vi "SentinelController v35 good v11.vi"() -> ()   [LabVIEW 2011]
uses:
  SC MT99XX tester states.ctl
  SC handler states.ctl
  Handler Types.ctl
  SC NS6040 tester states.ctl
  Echo tester states.ctl
  <vilib>/Instr/_visa.llb/Select Event Type.ctl
  <userlib>/configTool/configTool.llb/initConfigGlobal.vi
  <userlib>/configTool/configTool.llb/loadConfigFile.vi
  <userlib>/configTool/configTool.llb/closeConfig.vi
  <userlib>/configTool/configTool.llb/getProperty(DBL).vi
  <userlib>/configTool/configTool.llb/getProperty(U32).vi
  <userlib>/configTool/configTool.llb/getProperty(BOOL).vi
  <userlib>/configTool/configTool.llb/getProperty(I32).vi
  <userlib>/configTool/configTool.llb/getProperty(STR).vi
panel:
  out "Numeric 4":i32
  out "Numeric 3":i32
  out "Numeric 2":i32
  out "Numeric":i32
  out "H2 wt start hidden":u32
  out "H2 wt end hidden":u32
  out "H2 it start hidden":u32
  out "H2 it end hidden":u32
  out "H2 tt start hidden":u32
  out "H2 tt end hidden":u32
  in  "Data log path and filename":path=path "configuraitons/default_configuraiton.cfg"
  in  "Panels":T1(tab)=enum."System Configuration"
  in  "Test cell ID":string="default"
  in  "Operator name":string="default"
  in  "Lot number":string="default"
  in  "Configuration file path and filename":path
  in  "POWER":bool=TRUE
  in  "Tester Handler Config":T2=enum."Seiko-Epson NS6040" caption="Handler type"
  in  "H1 handler type":T2=enum."Seiko-Epson NS6040" caption="Handler type"
  in  "H2 handler type":T2=enum."Seiko-Epson NS6040" caption="Handler type"
  in  "H2 allow lower parallelism":bool
  in  "H1 allow lower parallelism":bool
  in  "H1 low yield warning":dbl=95.0 min=0.0 max=100.0 step=1.0
  in  "Ignore alarms until AFTER this many cycles":i32=20
  in  "H1 low yield alarm":dbl=85.0 min=0.0 max=100.0 step=1.0
  in  "H1 low UPH warning (%)":dbl=95.0 min=1.0 max=48000.0 step=1.0
  in  "H1 low UPH alarm (%)":dbl=90.0 min=1.0 max=48000.0 step=1.0
  in  "Enable data logging of all events":bool=TRUE
  in  "Enable electronic notification of alarms":bool
  in  "H2 low UPH alarm (%)":dbl=90.0 min=1.0 max=48000.0 step=1.0
  in  "H2 low UPH warning (%)":dbl=95.0 min=1.0 max=48000.0 step=1.0
  in  "H2 low yield alarm":dbl=90.0 min=0.0 max=100.0 step=1.0
  in  "H2  low yield warning":dbl=95.0 min=0.0 max=100.0 step=1.0
  in  "H1 enable halt\non yield alarm":bool
  in  "H2 enable halt\non yield alarm":bool
  in  "H1 enable halt\non UPH alarm":bool
  in  "H2 enable halt\non UPH alarm":bool
  out "H2 Device Count":u32 caption="Device Count"
  out "H1 Device Count":u32 caption="Decvice Count"
  out "H1 Good Units":u32 caption="Decvice Count"
  out "H2 Good Units":u32 caption="Device Count"
  out "H1 lot yield mon":dbl format="%.1f"
  out "H2 lot yield mon":dbl format="%.1f"
  out "UPH averaging":u32=20 min=2 max=100 step=1
  out "Yield averaging":u32=20 min=2 max=100 step=1
  in  "Push to reset charts":bool
  in  "Run":bool caption="Run / Stop"
  in  "Optimize handler speed":bool
  out "H1 parallelism":u32
  out "Utilization averaging":i32=6 min=2 max=20 step=1
  out "H2 nominal 2":bool=TRUE
  out "H2 warning 2":bool
  out "H2 alarm 2":bool
  out "H1 nominal 2":bool=TRUE
  out "H1 warning 2":bool
  out "H1 alarm 2":bool
  out "H2 nominal":bool=TRUE
  out "H2 warning":bool
  out "H2 alarm":bool
  out "H1 nominal":bool=TRUE
  out "H1 warning":bool
  out "H1 alarm":bool
  out "H2 Lock":bool
  out "H1 Lock":bool
  out "H2 measured Test Time":dbl caption="Index Time" format="%.2f"
  out "H2 measured  Index Time":dbl caption="Index Time" format="%.2f"
  out "H2 Indexing":bool
  out "H2 Testing":bool
  out "H2 Ready with sites":bool
  out "H2 On/Off-line":bool
  out "H2 measured Wait Time":dbl caption="Index Time" format="%.2f"
  out "H1 measured Test Time":dbl caption="Index Time" format="%.2f"
  out "H1 measured Index Time":dbl caption="Index Time" format="%.2f"
  out "H1 Indexing":bool
  out "H1 Testing":bool
  out "H1 Ready with sites":bool
  out "H1 On/Off-line":bool
  out "H1 measured Wait Time":dbl caption="Index Time" format="%.2f"
  out "System UPH":u32(knob) caption="Sys UPH" scale=0.0..30240.0 scale format="%#.0f"
  out "H2 UPH":cluster{u32, u32}(knob) scale=0.0..14400.0 scale format="%#.0f"
  out "H1 UPH":cluster{u32, u32}(knob) scale=0.0..14400.0 scale format="%#.0f"
  out "Sys utilization":dbl(knob) caption="Yield" scale=0.0..100.0
  in  "H2 online":bool=TRUE
  in  "H1 online":bool=TRUE
  in  "Tester online":bool=TRUE
  in  "Alert volume":u32(knob)=5 max=10 step=1 scale=0.0..10.0
  in  "Audio On / Off":bool
  out "SysUtilMon":cluster{i32, i32}(graph)
  out "H2 parallelism":u32 caption="H2 Paralellism"
  out "YieldMon":cluster{i32, i32, i32, i32}(graph)
  out "Program Parallelism":u32=8 caption="Tester Parallelism" min=1 max=16 step=1
  out "H2 calc UPH":dbl format="%#.0f"
  out "H1 Index Time 2":dbl caption="H1 index time"
  out "H1 Test Time 2":dbl caption="H1 test time"
  out "H1 P in formula":u32 caption="H1 Parallelism"
  out "H2 UPH per unit area":dbl format="%.1f"
  out "H1 calc UPH":dbl format="%#.0f"
  out "H1 UPH per unit area":dbl format="%.1f"
  out "Std mo cost ($/mo)":dbl
  out "Std unit cost\n(cents/device)":dbl format="%.3g"
  out "UPH":dbl format="%#.0f"
  in  "Hours per month":i32=730
  out "Std hourly\ncost ($/hr)":dbl format="%.2f"
  in  "Std cell \nfloorspace area":i32=200 min=10 max=1000 step=10
  in  "Overhead ($/mo)":dbl=1000.0 min=0.0 max=10000.0 step=100.0
  in  "Handler cost ($/mo)":dbl=2500.0 min=0.0 max=100000.0 step=100.0
  in  "Tester cost ($/mo)":dbl=8500.0 min=0.0 max=100000.0 step=500.0
  in  "Utilization (%)":u32=80 min=10 max=100 step=10
  out "Calendar days required\nfor testing all units":dbl format="%.1f"
  in  "# of devices to test":u32=10000000 min=1000 max=100000000 step=1000
  out "$ saved":i64 format="%#.0f"
  out "H2 IT (scycle)":dbl format="%.2f"
  out "H2 TT (s/cycle)":dbl format="%.2f"
  out "H2 WT (s/cycle)":dbl format="%.2f"
  out "H1 WT (s/cycle)":dbl format="%.2f"
  out "H1 IT (s/cycle)":dbl format="%.2f"
  out "H1 TT (s/cycle)":dbl format="%.2f"
  out "H2 units/cycle":u32 caption="H1 Parallelism"
  out "H1 units/cycle":u32
  out "Calc H1 UPH":u32
  out "Calc H2 UPH":u32
  out "Std cell floorspace area":i32
  out "Tandem unit cost\n(cents/device)":dbl format="%.3f"
  out "Hours per month 2":i32 caption="Hours per month"
  out "Total Mo Costs ($/mo) 3":dbl caption="Tandem mo cost ($/mo)"
  out "Total Mo Costs ($/mo) 2":dbl caption="Std mo cost ($/mo)"
  out "Calc\nsystem UPH":u32 caption="Simulated\nSystem UPH"
  out "Tandem\nfloorspace area":i32
  out "Tandem UPH\nper unit area":dbl format="%.1f"
  in  "Second handler cost ($/mo)":dbl=2500.0 min=0.0 max=10000.0 step=100.0
  out "Tandem hourly\ncost ($/hr)":dbl format="%.2f"
  in  "Celerint licensing cost ($/mo)":dbl=1000.0 min=0.0 max=10000.0 step=100.0
  in  "Celerint hardware cost ($/mo)":dbl min=0.0 max=10000.0 step=1.0
  in  "Additional floorspace\nfor second handler":i32=50 min=0 max=1000 step=10
  out "Number of text alerts":u32 caption="Number of alerts\nsent as notifications"
  in  "Enable text notification":bool
  out "Notifications Lot Display":string="default" caption="Lot number (not editable)"
  in  "Include\ndata log as\nattachment":bool=TRUE
  out "Number of email alerts":u32 caption="Number of alerts\nsent as notifications"
  out "Email alert - attachment (not editable)":path
  in  "Email alert - message":string="An alarm event has ocurred on a semiconductor test lot that you have requested to monitor.  Please see the attached data log for event details.\n\nThis message is generated automatically by the Sentinel Controller program.\n\nTo stop these messages, please contact the test floor operator and disable automatic alert notifictions.\n\n"
  in  "Email alert - engineer":string="harry@celerint.com"
  in  "Email alert - CC":string="hjr@celerint.com"
  in  "Enable email notification":bool
  in  "Carrier":enum16{"T-Mobile", "AT&T", "Verizon", "Sprint"}(ring)=enum."AT&T"
  in  "Phone number":string="5128263411"
  in  "Subject":string="From: Sentinel Controller"
  in  "Body":string="An alarm event has ocurred"
  in  "GPIB wait time (ms)":u32=1000
  in  "Slow for  Diagnostics":bool=TRUE
  out "GPIB bus 0 read error":bool
  out "GPIB Bus 0 traffic":string
  out "GPIB bus 1 traffic":string
  out "GPIB bus 2 traffic":string
  out "GPIB bus 0 write error":bool
  out "GPIB bus 1 read error":bool
  out "GPIB bus 1 write error":bool
  out "GPIB bus 2 write error":bool
  out "GPIB bus 2 read error":bool
  out "VISA bus 1 open error":bool
  out "VISA bus 2 open error":bool
  out "VISA bus 0 open error":bool
  out "VISA bus 0 close error":bool
  out "VISA bus 1 close error":bool
  out "VISA bus 2 close error":bool
  out "Decrease Handler Velocity":string
  out "Increase Handler Velocity":string
  out "Get Handler Velocity":string
  in  "SentCtrl listens to tester at":refnum<visa-resource-name>="GPIB0::INTFC"
  out "H2 Address":string
  out "H1 Address":string
  out "Tester address":string
  in  "SentCtrl talks to tester at":refnum<visa-resource-name>="GPIB0::0::INSTR"
  in  "SentCtrl listens to handler 1 at":refnum<visa-resource-name>="GPIB1::INTFC"
  in  "SentCtrl talks to handler 1 at":refnum<visa-resource-name>="GPIB1::1::INSTR"
  in  "SentCtrl listens to handler 2 at":refnum<visa-resource-name>="GPIB2::INTFC"
  in  "SentCtrl talks to handler 2 at":refnum<visa-resource-name>="GPIB2::1::INSTR"
  in  "Ni Logo":bool
  in  "Ni Logo 2":bool
  in  "Echo state of tester hid":T3
  in  "H1 echo hid":string
  in  "H2 echo hid":string
  in  "SRQ MASK from tester hid":string
  in  "H1 binning string hid":string
  in  "H2 binning string hid":string
  in  "H1 FULLSITES? response hid":string
  in  "H2 FULLSITES? response hid":string
  in  "H1 FULLSITES? binary hid":string
  in  "H2 FULLSITES? binary hid":string
  in  "H1 response to SPOLL hid":string
  in  "H2 response to SPOLL hid":string
  in  "H1 response to FR? hid":string
  in  "H2 response to FR? hid":string
  in  "NS6040 tester states H1 hid":T4
  in  "NS6040 tester states H2 hid":T4
  in  "MT99XX tester states H2 hid":T5
  in  "MT99XX tester states H1 hid":T5
  in  "GPIB parsed msg from tester hid":string
  in  "Message from H2 hid":string
  in  "Message from H1 hid":string
  in  "Message from tester hid":string
  in  "H1 response to *IDN? hid":string
  in  "H2 response to *IDN? hid":string
  in  "GPIB wait timeout hid":u32
  out "Number of data log entries hid":u32
  in  "Last locked handler hid":enum16{"H1", "H2"}(ring)
  out "SC measured wait time hid":dbl
  out "Exit SC tester H2 StMach hid":bool
  out "Exit SC tester H1 StMach hid":bool
  out "Exit SC handler StMach hid":bool
  out "H2 response to *HAND? hid":string
  out "H1 response to *HAND? hid":string
  in  "Tester loop counter hid":u32
  in  "H2 loop counter hid":u32
  in  "H1 loop counter hid":u32
  in  "Test Cycle State hid":T6(ring)
  in  "Test time expected hid":dbl
  out "H1 it end hidden":u32
  out "H1 wt start hidden":u32
  out "H1 tt start hidden":u32
  out "H1 wt end hidden":u32
  out "H1 tt end hidden":u32
  out "H1 it start hidden":u32
  in  "H1 SITES? response hid":string
  out "VISA bus 1 resource name out hid":refnum<visa-resource-name>
  out "VISA bus 1 error out hid":errorcluster
  out "VISA bus 2 error out hid":errorcluster
  out "VISA bus 2 resource name out hid":refnum<visa-resource-name>
  out "VISA bus 0 error out hid":errorcluster
  out "tester wt start hid":u32
  out "tester wt end hid":u32
  out "tester tt start hid":u32
  out "tester tt end hid":u32
  out "SC measured test time hid":dbl
  in  "Binning string from tester hid":string
  out "VISA bus 0 resource name out hid":refnum<visa-resource-name>
  in  "SC handler states hid":T7
  out "H1 Single Handler UPH hid":dbl
  out "H1 UPH warning limit hid":dbl
  out "H1 UPH alarm limit hid":dbl
  out "H2 Single Handler UPH hid":dbl
  out "H2 UPH warning limit hid":dbl
  out "H2 UPH alarm limit hid":dbl
  in  "Min Test Time hid":dbl=0.499 caption="Min Test Time" min=0.1 max=1.0 step=0.1 format="%#.1g"
  in  "H2 index time expected hid":dbl
  in  "H1 index time expected hid":dbl
  in  "system states hid":T8(ring)
  in  "system statuts hid":T9(ring)
  out "H1 cycle yield hid":dbl format="%.1f"
  out "H2 cycle yield hid":dbl format="%.1f"
  in  "H2 SITES? response hid":string
  # "Sentinel Controller\nfor\nTandlem Handler\nTest Cells \nwww.celerint.com"
  # "Turning off POWER will stop execution the Sentinel Controller Program"
  # "INPUT FILE"
  # "LOT INFORMATION"
  # "Celerint Sentinel Controller"
  # "SYSTEM SETTINGS"
  # "Tester Handler Config"
  # "Handler  1"
  # "Handler 2"
  # "Set UPH thresholds as % of max UPH"
  # "Set UPH thresholds as % of max UPH"
  # "test cycles (insertions)"
  # "Celerint Sentinel Controller"
  # "Handler 2"
  # "Handler 1"
  # "Yield"
  # "UPH"
  # "Yield"
  # "UPH"
  # "parallelism"
  # "lot yield (%)"
  # "good devices"
  # "devices tested"
  # "Data"
  # "Avg"
  # "wait time"
  # "index time"
  # "test time"
  # "waiting"
  # "H1"
  # "H2"
  # "testing"
  # "indexing"
  # "on/off-line"
  # "STANDARD SETUP"
  # "H2 calculated\nsimilarly"
  # "3600"
  # "Celerint Sentinel\nController Simulator"
  # "TANDEM HANDLER SETUP"
  # "SAVINGS"
  # "3600 (s/hr)"
  # "3600 (s/hr)"
  # "Celerint Sentinel Controller"
  # "Lot number will be appended automatically:"
  # "This data is read from the INI file (.cfg)\nat program start and is used to configure\nthe various GPIB interfaces on the Sentinel\nController."
  # "These setting are created based on the addresses read from the INI file."
  # "Laptop Tester Sim\nGPIB0,SC\naddress 0\nlisten at: GPIB0::INTFC\ntalk to: GPIB0::1::INSTR"
  # "*SITES?"
  # "binning"
  # "Bus 0"
  # "1011"
  # "SC\nGPIB0,Non-SC\naddress 1\nlisten at: GPIB0::INTFC\ntalk to: GPIB0::0::INSTR"
  # "SC\nGPIB1,SC\naddress 0\nlisten at: GPIB1::INTFC\ntalk to: GPIB1::0::INSTR"
  # "SC\nGPIB2,SC\naddress 0\nlisten at: GPIB2::INTFC\ntalk to: GPIB2::0::INSTR"
  # "NI PXI-1031"
  # "*SITES?"
  # "binning"
  # "*SITES?"
  # "binning"
  # "Bus 1"
  # "Bus 2"
  # "1011"
  # "1011"
  # "Laptop H1 Sim\nGPIB1,Non-SC\naddress 1\nlisten at: GPIB1::INTFC\ntalk to: GPIB1::0::INSTR"
  # "Laptop H2 Sim\nGPIB2,Non-SC\naddress 1\nlisten at: GPIB2::INTFC\ntalk to: GPIB2::0::INSTR"
  # "Note:\nUsually, there are default GPIB addresses used for the tester and handler.\nThese addresses are read in from the INI file (.cfrg extension) when this\nprogram initializes.  For the purposes of this map, we are using  these defaults:\n          - Semiconductor tester default GPIB address: 6\n          - Semiconductor handler default GPIB address: 14\nFor the purposes of this illustration, these addresses are purely arbitrary."
  # "Tester\nGPIB0,SC\naddress 6\nlisten at: GPIB0::INTFC\ntalk to: GPIB0:14::INSTR"
  # "*SITES?"
  # "binning"
  # "Bus 0"
  # "1011"
  # "SC\nGPIB0,Non-SC\naddress 14\nlisten at: GPIB1::INTFC\ntalk to: GPIB1:6::INSTR"
  # "SC\nGPIB1,SC\naddress 6\nlisten at: GPIB1::INTFC\ntalk to: GPIB1:14::INSTR"
  # "SC\nGPIB2,SC\naddress 6\nlisten at: GPIB2::INTFC\ntalk to: GPIB2:14::INSTR"
  # "NI PXI-1031"
  # "*SITES?"
  # "binning"
  # "*SITES?"
  # "binning"
  # "Bus 1"
  # "Bus 2"
  # "1011"
  # "1011"
  # "Handler 1\nGPIB0,Non-SC\naddress 14\nlisten at: GPIB0::INTFC\ntalk to: GPIB0:6::INSTR"
  # "Handler 2\nGPIB0,Non-SC\naddress 14\nlisten at: GPIB0::INTFC\ntalk to: GPIB0:6::INSTR"
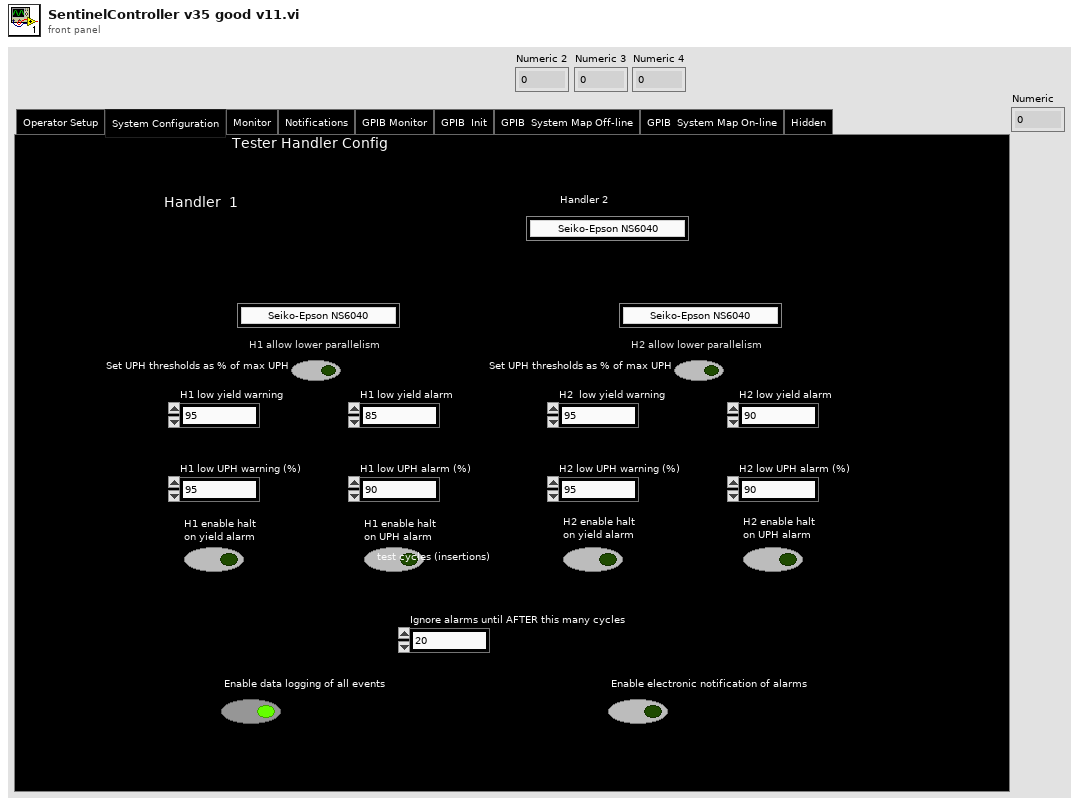
[diagram p1: front panel]
types:
  T1 = enum32{"Operator Setup", "System Configuration", "Monitor", "Benefit Analysis", "Notifications", "GPIB Monitor", "GPIB  Init", "GPIB  System Map Off-line", "GPIB  System Map On-line", "Hidden"}
  T2 = typedef "Handler Types.ctl" = enum16{"Multitest", "Seiko-Epson NS6040"}
  T3 = typedef "Echo tester states.ctl" = enum16{"ECHONG", "ECHOOK", "NO ECHO"}
  T4 = typedef "SC NS6040 tester states.ctl" = enum16{"initializing bus", "sending *IDN?", "serial polling handler", "sending Fullsites?", "testing", "sending BINON?", "sending ECHONG", "sending ECHOOK", "closing bus"}
  T5 = typedef "SC MT99XX tester states.ctl" = enum16{"initializing bus", "polling *SITES?", "sending *IDN?", "testing", "binning", "closing bus"}
  T6 = enum16{"idled", "SOT received", "SOT sent", "binning sent", "binning received", "sites ready received", "sites ready sent"}
  T7 = typedef "SC handler states.ctl" = enum16{"initializing bus", "waiting on event", "waiting on serial poll", "reading", "responding to *IDN?", "responding to Fullsites?", "responding to SITES?", "responding to HIDN?", "respond to HAND?", "testing", "responding to BINON", "responding to A BIN", "ECHONG", "ECHOOK", "responding to unknown command", "closing bus"}
  T8 = enum16{"H1 Ready", "H2 Ready", "No Handler Ready"}
  T9 = enum16{"H1NH2N", "H1NH2W", "H1NH2A", "H1WH2N", "H1WH2W", "H1WH2A", "H1AH2N", "H1AH2W", "H1AH2A"}
  T10 = enum16{"open", "replace", "create", "open or create", "replace or create", "replace or create with confirmation"}
  T11 = typedef "configRef.ctl" = refnum<vi>
  T12 = cluster{i32, "rolling avg out":dbl, "H1 low yield alarm":dbl, "H2 low yield alarm":dbl}
  T13 = cluster{"rolling avg out":dbl, i32, "H1 low yield alarm":dbl, "H2 low yield alarm":dbl}
  T14 = typedef "Select Event Type.ctl" = u32
diagram:
  n1 = flat-sequence {
    frame #0 {
      # "This frame contains ALL declarations for control and indicators.\nAll hidden objects are on frame #9.  On the front panel, these hidden\nobjects are located on a tab that is hidden."
      n2 = stacked-sequence {
        frame #0 {
        }
        frame #1 {
          # "Operator Setup Tab"
        }
        frame #2 {
          # "System Config Tab"
        }
        frame #3 {
          w2 = FALSE ("H2 Testing")
          w1 = FALSE ("H1 Testing")
          # "Monitor Tab"
          n3 = local write "Run"(FALSE ("Run")) -> ()
          "H1 Testing" <- w1
          "H1 Ready with sites" <- w1
          "H1 Indexing" <- w1
          "H2 Testing" <- w2
          "H2 Ready with sites" <- w2
          "H2 Indexing" <- w2
          "H2 Good Units" <- 0
          "H2 Device Count" <- 0
          "H2 lot yield mon" <- 100.0 ("H2 Yield  Mon")
          "H1 lot yield mon" <- 100.0 ("H1 Yield Mon")
          "H1 Good Units" <- u32 0
          "H1 Device Count" <- u32 0
        }
        frame #4 {
          # "Benefits Tab"
        }
        frame #5 {
          # "Notifications"
        }
        frame #6 {
          # "GPIB Monitor"
          n4 = local write "Slow for  Diagnostics"(FALSE ("Slow for  Diagnostics")) -> ()
          n5 = local write "GPIB wait time (ms)"(u32 1000 ("GPIB wait time (ms)")) -> ()
        }
        frame #7 {
          # "GPIB Init"
        }
        frame #8 {
          # "GPIB System Maps - Bothg off-line and on-line combined"
        }
        frame #9 {
          (unwired) 0.031 ("tester measured wait time")
          # "Hidden controls and indicators"
          n6 = local write "Last locked handler hid"(enum16{"H1", "H2"}."H1" ("Last locked handler")) -> ()
          "SC measured test time hid" <- 1.0 ("tester measured test time")
          "H1 response to *HAND? hid" <- "" ("H1 response to *HAND? hidden")
          "H2 response to *HAND? hid" <- "" ("H2 response to *HAND? hidden")
          "Exit SC handler StMach hid" <- FALSE ("Exit tester state machine")
          "Exit SC tester H1 StMach hid" <- FALSE ("Exit H1 state machine")
          "Exit SC tester H2 StMach hid" <- FALSE ("Exit H2 state machine")
          "SC measured wait time hid" <- 1.0 ("tester measured wait time hid")
          "H2 cycle yield hid" <- 100.0 ("H2 Yield  Mon")
          "H1 cycle yield hid" <- 100.0 ("H1 Yield Mon")
        }
      }
    }
    frame #1 {
      n7 = local write "POWER"(TRUE ("POWER")) -> ()
    }
    frame #2 {
      # "This frame handles verifying that the configuration file exists and is valaid.\nIt also creates the data log."
      n8 = local read "Configuration file path and filename"() -> (w25:path)
      n9 = call <vilib>:"Application Directory.vi"() -> ("Application Directory"=w27:path)
      n10 = Equal?(x=w25, y=path "") -> (x = y?=w24:bool)
      n11 = Get Date/Time String(want seconds? (F)=TRUE) -> (date string=w40:string, time string=w32:string)  [unwired: 2 in]
      n12 = Build Path(base path=w27, name or relative path="datalogs") -> (appended path=w45:path)
      n13 = Path To String(path=w45) -> (string=w36:string)
      n14 = Search and Replace String(replace all?=TRUE ("replace all? (F)"), input string=w40, search string="/", replace string="-" ("replace string (\"\")")) -> (result string=w30:string)  [unwired: 4 in, 3 out]
      n15 = Search and Replace String(replace all?=TRUE ("replace all? (F)"), input string=w32, search string=":", replace string="." ("replace string (\"\")")) -> (result string=w31:string)  [unwired: 4 in, 3 out]
      n16 = case shown="True" w24 {
        tunnel: w25 -> [w47 _]
        frame False {
          n17 = call <vilib>:"Check if File or Folder Exists.vi"("path"=w47) -> ("file or folder exists?"=w46:bool)  [unwired: 8 in, 2 out]
          n18 = case shown="False" w46 {
            frame False {
              n19 = local write "POWER"(FALSE ("POWER")) -> ()
              n20 = One Button Dialog(message="Fatal error 100: \nConfiguration file does not exist!", button name ("OK")="Dismiss and Restart") -> ()  [unwired: 1 out]
            }
            frame True {
              n21 = local read "Configuration file path and filename"() -> (w54:path)
              n22 = call-poly <userlib>:"manageConfig.vi"() -> ("config ref out"=w55:T11)  [unwired: 10 in, 1 out]
              n23 = call-poly <userlib>:"manageConfig.vi"("access (0:read/write)"=enum16{"read/write", "read-only", "write-only"}."read-only", "config file path"=w54, "config ref"=w55) -> ("error out"=w53:errorcluster, "config ref out"=w51:T11)  [unwired: 6 in, 1 out]
              n24 = Unbundle By Name(w53) -> ("status"=w52:bool)
              n25 = call-poly <userlib>:"manageConfig.vi"("config ref"=w51) -> ()  [unwired: 10 in, 1 out]
              n26 = case shown="True" w52 {
                frame False {
                }
                frame True {
                  n27 = local write "POWER"(FALSE ("POWER")) -> ()
                  n28 = One Button Dialog(message="Fatal error 101:\nConfiguration file is corrupted\nor is not a compliant format!", button name ("OK")="Dismiss and Restart") -> ()  [unwired: 1 out]
                }
              }
            }
          }
        }
        frame True {
          n29 = call <vilib>:"Application Directory.vi"() -> ("Application Directory"=w63:path)
          n30 = Build Path(base path=w63, name or relative path="configurations") -> (appended path=w60:path)
          n31 = Path To String(path=w60) -> (string=w65:string)
          n32 = Concatenate Strings(w65, "\\" ("string"), "default_configuration.cfg" ("string")) -> (w66:string)
          n33 = String To Path(string=w66) -> (path=w67:path)
          n34 = local write "Configuration file path and filename"(w67) -> ()
        }
      }
      n35 = Concatenate Strings(w36, "\\" ("string"), w30, " " ("string"), w31, ".txt" ("string")) -> (w42:string)
      n36 = String To Path(string=w42) -> (path=w44:path)
      n37 = local write "Data log path and filename"(w44) -> ()
    }
    frame #3 {
      # "This frame reads the INI file and initializes all data that is under engineering control."
      n38 = local read "POWER"() -> (w68:bool)
      n39 = case shown="True" w68 {
        frame False {
        }
        frame True {
          n40 = stacked-sequence {
            frame #0 {
              # "Load data from the INI file for the System Configuration tab"
              n41 = local read "Configuration file path and filename"() -> (w162:path)
              n42 = call-poly <userlib>:"manageConfig.vi"() -> ("config ref out"=w163:T11)  [unwired: 10 in, 1 out]
              n43 = call-poly <userlib>:"manageConfig.vi"("access (0:read/write)"=enum16{"read/write", "read-only", "write-only"}."read-only", "config file path"=w162, "config ref"=w163) -> ("error out"=w101:errorcluster, "config ref out"=w100:T11)  [unwired: 6 in, 1 out]
              n44 = call-poly <userlib>:"manageConfig.vi"("error in"=w101, "property path"="SCS.SimCfgCtrls.Test time expected" ("key"), "config ref"=w100) -> ("error out"=w97:errorcluster, "data"=w103:dbl, "config ref out"=w104:T11)  [unwired: 5 in, 1 out]
              n45 = local write "Test time expected hid"(w103) -> ()
              n46 = call-poly <userlib>:"manageConfig.vi"("error in"=w97, "property path"="SCS.SimCfgCtrls.H1 Parallelism", "config ref"=w104) -> ("error out"=w96:errorcluster, "value"=w116:u32, "config ref out"=w110:T11)  [unwired: 5 in, 1 out]
              n47 = local write "H1 parallelism"(w116) -> ()
              n48 = call-poly <userlib>:"manageConfig.vi"("error in"=w96, "property path"="SCS.SimCfgCtrls.H2 Parallelism", "config ref"=w110) -> ("error out"=w95:errorcluster, "value"=w112:u32, "config ref out"=w109:T11)  [unwired: 5 in, 1 out]
              n49 = local write "H2 parallelism"(w112) -> ()
              n50 = call-poly <userlib>:"manageConfig.vi"("error in"=w95, "property path"="SCS.SimCfgCtrls.Program Parallelism", "config ref"=w109) -> ("error out"=w94:errorcluster, "value"=w111:u32, "config ref out"=w102:T11)  [unwired: 5 in, 1 out]
              n51 = local write "Program Parallelism"(w111) -> ()
              n52 = call-poly <userlib>:"manageConfig.vi"("error in"=w94, "property path"="SCS.SimCfgCtrls.H1 index time expected", "config ref"=w102) -> ("error out"=w93:errorcluster, "data"=w106:dbl, "config ref out"=w115:T11)  [unwired: 5 in, 1 out]
              n53 = local write "H1 index time expected hid"(w106) -> ()
              n54 = call-poly <userlib>:"manageConfig.vi"("error in"=w93, "property path"="SCS.SimCfgCtrls.H2 index time expected", "config ref"=w115) -> ("error out"=w99:errorcluster, "data"=w105:dbl, "config ref out"=w98:T11)  [unwired: 5 in, 1 out]
              n55 = local write "H2 index time expected hid"(w105) -> ()
              n56 = call-poly <userlib>:"manageConfig.vi"("error in"=w99, "property path"="SCS.SimCfgCtrls.H1 low yield warning" ("key"), "config ref"=w98) -> ("error out"=w92:errorcluster, "data"=w139:dbl, "config ref out"=w149:T11)  [unwired: 5 in, 1 out]
              n57 = local write "H1 low yield warning"(w139) -> ()
              n58 = call-poly <userlib>:"manageConfig.vi"("error in"=w92, "property path"="SCS.SimCfgCtrls.H1 low yield alarm", "config ref"=w149) -> ("error out"=w91:errorcluster, "data"=w138:dbl, "config ref out"=w148:T11)  [unwired: 5 in, 1 out]
              n59 = local write "H1 low yield alarm"(w138) -> ()
              n60 = call-poly <userlib>:"manageConfig.vi"("error in"=w91, "property path"="SCS.SimCfgCtrls.H1 low UPH warning (%)", "config ref"=w148) -> ("error out"=w90:errorcluster, "data"=w137:dbl, "config ref out"=w150:T11)  [unwired: 5 in, 1 out]
              n61 = local write "H1 low UPH warning (%)"(w137) -> ()
              n62 = call-poly <userlib>:"manageConfig.vi"("error in"=w90, "property path"="SCS.SimCfgCtrls.H1 low UPH alarm (%)", "config ref"=w150) -> ("error out"=w89:errorcluster, "data"=w136:dbl, "config ref out"=w151:T11)  [unwired: 5 in, 1 out]
              n63 = local write "H1 low UPH alarm (%)"(w136) -> ()
              n64 = call-poly <userlib>:"manageConfig.vi"("error in"=w89, "property path"="SCS.SimCfgCtrls.H1 enable halt on yield alarm", "config ref"=w151) -> ("error out"=w88:errorcluster, "value"=w135:bool, "config ref out"=w152:T11)  [unwired: 5 in, 1 out]
              n65 = local write "H1 enable halt\non yield alarm"(w135) -> ()
              n66 = call-poly <userlib>:"manageConfig.vi"("error in"=w88, "property path"="SCS.SimCfgCtrls.H1 enable halt on UPH alarm", "config ref"=w152) -> ("error out"=w87:errorcluster, "value"=w134:bool, "config ref out"=w153:T11)  [unwired: 5 in, 1 out]
              n67 = local write "H1 enable halt\non UPH alarm"(w134) -> ()
              n68 = call-poly <userlib>:"manageConfig.vi"("error in"=w87, "property path"="SCS.SimCfgCtrls.H2 low yield warning", "config ref"=w153) -> ("error out"=w86:errorcluster, "data"=w133:dbl, "config ref out"=w154:T11)  [unwired: 5 in, 1 out]
              n69 = local write "H2  low yield warning"(w133) -> ()
              n70 = call-poly <userlib>:"manageConfig.vi"("error in"=w86, "property path"="SCS.SimCfgCtrls.H2 low yield alarm", "config ref"=w154) -> ("error out"=w85:errorcluster, "data"=w132:dbl, "config ref out"=w155:T11)  [unwired: 5 in, 1 out]
              n71 = local write "H2 low yield alarm"(w132) -> ()
              n72 = call-poly <userlib>:"manageConfig.vi"("error in"=w85, "property path"="SCS.SimCfgCtrls.H2 low UPH warning (%)", "config ref"=w155) -> ("error out"=w84:errorcluster, "data"=w131:dbl, "config ref out"=w123:T11)  [unwired: 5 in, 1 out]
              n73 = local write "H2 low UPH warning (%)"(w131) -> ()
              n74 = call-poly <userlib>:"manageConfig.vi"("error in"=w84, "property path"="SCS.SimCfgCtrls.H2 low UPH alarm (%)", "config ref"=w123) -> ("error out"=w83:errorcluster, "data"=w121:dbl, "config ref out"=w122:T11)  [unwired: 5 in, 1 out]
              n75 = local write "H2 low UPH alarm (%)"(w121) -> ()
              n76 = call-poly <userlib>:"manageConfig.vi"("error in"=w83, "property path"="SCS.SimCfgCtrls.H2 enable halt on yield alarm", "config ref"=w122) -> ("error out"=w82:errorcluster, "value"=w130:bool, "config ref out"=w156:T11)  [unwired: 5 in, 1 out]
              n77 = local write "H2 enable halt\non yield alarm"(w130) -> ()
              n78 = call-poly <userlib>:"manageConfig.vi"("error in"=w82, "property path"="SCS.SimCfgCtrls.H2 enable halt on UPH alarm", "config ref"=w156) -> ("error out"=w81:errorcluster, "value"=w129:bool, "config ref out"=w120:T11)  [unwired: 5 in, 1 out]
              n79 = local write "H2 enable halt\non UPH alarm"(w129) -> ()
              n80 = call-poly <userlib>:"manageConfig.vi"("error in"=w81, "property path"="SCS.SimCfgCtrls.Ignore alarms until this many cycles", "config ref"=w120) -> ("error out"=w80:errorcluster, "value"=w128:i32, "config ref out"=w119:T11)  [unwired: 5 in, 1 out]
              n81 = local write "Ignore alarms until AFTER this many cycles"(w128) -> ()
              n82 = call-poly <userlib>:"manageConfig.vi"("error in"=w80, "property path"="SCS.SimCfgCtrls.Enable data logging", "config ref"=w119) -> ("error out"=w79:errorcluster, "value"=w127:bool, "config ref out"=w140:T11)  [unwired: 5 in, 1 out]
              n83 = local write "Enable data logging of all events"(w127) -> ()
              n84 = call-poly <userlib>:"manageConfig.vi"("error in"=w79, "property path"="SCS.SimCfgCtrls.Enable electronic notification of alarms", "config ref"=w140) -> ("error out"=w78:errorcluster, "value"=w126:bool, "config ref out"=w76:T11)  [unwired: 5 in, 1 out]
              n85 = local write "Enable electronic notification of alarms"(w126) -> ()
              n86 = call-poly <userlib>:"manageConfig.vi"("error in"=w78, "property path"="SCS.SimCfgCtrls.H1 allow lower parallelism", "config ref"=w76) -> ("error out"=w77:errorcluster, "value"=w70:bool, "config ref out"=w75:T11)  [unwired: 5 in, 1 out]
              n87 = local write "H1 allow lower parallelism"(w70) -> ()
              n88 = call-poly <userlib>:"manageConfig.vi"("error in"=w77, "property path"="SCS.SimCfgCtrls.H2 allow lower parallelism", "config ref"=w75) -> ("error out"=w73:errorcluster, "value"=w69:bool, "config ref out"=w74:T11)  [unwired: 5 in, 1 out]
              n89 = local write "H2 allow lower parallelism"(w69) -> ()
              n90 = call-poly <userlib>:"manageConfig.vi"("error in (no error)"=w73, "config ref"=w74) -> ()  [unwired: 9 in, 1 out]
            }
            frame #1 {
              # "Load data from the INI file for the Monitor tab"
              n91 = local read "Configuration file path and filename"() -> (w201:path)
              n92 = call-poly <userlib>:"manageConfig.vi"() -> ("error out"=w175:errorcluster, "config ref out"=w202:T11)  [unwired: 10 in]
              n93 = call-poly <userlib>:"manageConfig.vi"("error in (no error)"=w175, "access (0:read/write)"=enum16{"read/write", "read-only", "write-only"}."read-only", "config file path"=w201, "config ref"=w202) -> ("error out"=w204:errorcluster, "config ref out"=w206:T11)  [unwired: 5 in, 1 out]
              n94 = call-poly <userlib>:"manageConfig.vi"("error in"=w204, "property path"="SCS.Monitor.Optimize handler speed" ("key"), "config ref"=w206) -> ("error out"=w174:errorcluster, "value"=w184:bool, "config ref out"=w176:T11)  [unwired: 5 in, 1 out]
              n95 = local write "Optimize handler speed"(w184) -> ()
              n96 = call-poly <userlib>:"manageConfig.vi"("error in"=w174, "property path"="SCS.Monitor.Tester on-line" ("key"), "config ref"=w176) -> ("error out"=w173:errorcluster, "value"=w183:bool, "config ref out"=w197:T11)  [unwired: 5 in, 1 out]
              n97 = local write "Tester online"(w183) -> ()
              n98 = call-poly <userlib>:"manageConfig.vi"("error in"=w173, "property path"="SCS.Monitor.H1 on-line" ("key"), "config ref"=w197) -> ("error out"=w172:errorcluster, "value"=w182:bool, "config ref out"=w196:T11)  [unwired: 5 in, 1 out]
              n99 = local write "H1 online"(w182) -> ()
              n100 = call-poly <userlib>:"manageConfig.vi"("error in"=w172, "property path"="SCS.Monitor.H2 on-line" ("key"), "config ref"=w196) -> ("error out"=w171:errorcluster, "value"=w181:bool, "config ref out"=w195:T11)  [unwired: 5 in, 1 out]
              n101 = local write "H2 online"(w181) -> ()
              n102 = call-poly <userlib>:"manageConfig.vi"("error in"=w171, "property path"="SCS.Monitor.Utilization averaging", "config ref"=w195) -> ("error out"=w170:errorcluster, "value"=w177:i32, "config ref out"=w194:T11)  [unwired: 5 in, 1 out]
              n103 = local write "Utilization averaging"(w177) -> ()
              n104 = call-poly <userlib>:"manageConfig.vi"("error in"=w170, "property path"="SCS.Monitor.Audio On/Off", "config ref"=w194) -> ("error out"=w169:errorcluster, "config ref out"=w193:T11)  [unwired: 5 in, 2 out]
              n105 = call-poly <userlib>:"manageConfig.vi"("error in"=w169, "property path"="SCS.Monitor.Alert volume", "config ref"=w193) -> ("error out"=w168:errorcluster, "value"=w180:u32, "config ref out"=w192:T11)  [unwired: 5 in, 1 out]
              n106 = local write "Alert volume"(w180) -> ()
              n107 = call-poly <userlib>:"manageConfig.vi"("error in"=w168, "property path"="SCS.Monitor.UPH averaging", "config ref"=w192) -> ("error out"=w167:errorcluster, "value"=w179:u32, "config ref out"=w191:T11)  [unwired: 5 in, 1 out]
              n108 = local write "UPH averaging"(w179) -> ()
              n109 = call-poly <userlib>:"manageConfig.vi"("error in"=w167, "property path"="SCS.Monitor.Yield averaging", "config ref"=w191) -> ("error out"=w166:errorcluster, "value"=w178:u32, "config ref out"=w190:T11)  [unwired: 5 in, 1 out]
              n110 = local write "Yield averaging"(w178) -> ()
              n111 = call-poly <userlib>:"manageConfig.vi"("error in (no error)"=w166, "config ref"=w190) -> ()  [unwired: 9 in, 1 out]
            }
            frame #2 {
              # "Load data from the INI file for the Benefits tab"
              n112 = local read "Configuration file path and filename"() -> (w243:path)
              n113 = call-poly <userlib>:"manageConfig.vi"() -> ("error out"=w216:errorcluster, "config ref out"=w244:T11)  [unwired: 10 in]
              n114 = call-poly <userlib>:"manageConfig.vi"("error in (no error)"=w216, "access (0:read/write)"=enum16{"read/write", "read-only", "write-only"}."read-only", "config file path"=w243, "config ref"=w244) -> ("error out"=w246:errorcluster, "config ref out"=w248:T11)  [unwired: 5 in, 1 out]
              n115 = call-poly <userlib>:"manageConfig.vi"("error in"=w246, "property path"="SCS.Benefits.Tester cost" ("key"), "config ref"=w248) -> ("error out"=w215:errorcluster, "data"=w234:dbl, "config ref out"=w225:T11)  [unwired: 5 in, 1 out]
              n116 = local write "Tester cost ($/mo)"(w234) -> ()
              n117 = call-poly <userlib>:"manageConfig.vi"("error in"=w215, "property path"="SCS.Benefits.Handler cost" ("key"), "config ref"=w225) -> ("error out"=w214:errorcluster, "data"=w233:dbl, "config ref out"=w224:T11)  [unwired: 5 in, 1 out]
              n118 = local write "Handler cost ($/mo)"(w233) -> ()
              n119 = call-poly <userlib>:"manageConfig.vi"("error in"=w214, "property path"="SCS.Benefits.Test cell overhead" ("key"), "config ref"=w224) -> ("error out"=w213:errorcluster, "data"=w232:dbl, "config ref out"=w223:T11)  [unwired: 5 in, 1 out]
              n120 = local write "Overhead ($/mo)"(w232) -> ()
              n121 = call-poly <userlib>:"manageConfig.vi"("error in"=w213, "property path"="SCS.Benefits.Hours per month" ("key"), "config ref"=w223) -> ("error out"=w212:errorcluster, "value"=w231:i32, "config ref out"=w222:T11)  [unwired: 5 in, 1 out]
              n122 = local write "Hours per month"(w231) -> ()
              n123 = call-poly <userlib>:"manageConfig.vi"("error in"=w212, "property path"="SCS.Benefits.STD cell floorspace area" ("key"), "config ref"=w222) -> ("error out"=w211:errorcluster, "value"=w230:i32, "config ref out"=w221:T11)  [unwired: 5 in, 1 out]
              n124 = local write "Std cell \nfloorspace area"(w230) -> ()
              n125 = call-poly <userlib>:"manageConfig.vi"("error in"=w211, "property path"="SCS.Benefits.Celerint hardware cost" ("key"), "config ref"=w221) -> ("error out"=w210:errorcluster, "data"=w229:dbl, "config ref out"=w220:T11)  [unwired: 5 in, 1 out]
              n126 = local write "Celerint hardware cost ($/mo)"(w229) -> ()
              n127 = call-poly <userlib>:"manageConfig.vi"("error in"=w210, "property path"="SCS.Benefits.Celerint licensing cost" ("key"), "config ref"=w220) -> ("error out"=w209:errorcluster, "data"=w228:dbl, "config ref out"=w219:T11)  [unwired: 5 in, 1 out]
              n128 = local write "Celerint licensing cost ($/mo)"(w228) -> ()
              n129 = call-poly <userlib>:"manageConfig.vi"("error in"=w209, "property path"="SCS.Benefits.Second handler cost" ("key"), "config ref"=w219) -> ("error out"=w208:errorcluster, "data"=w227:dbl, "config ref out"=w218:T11)  [unwired: 5 in, 1 out]
              n130 = local write "Second handler cost ($/mo)"(w227) -> ()
              n131 = call-poly <userlib>:"manageConfig.vi"("error in"=w208, "property path"="SCS.Benefits.Additional floorspace for seconed handler" ("key"), "config ref"=w218) -> ("error out"=w207:errorcluster, "value"=w226:i32, "config ref out"=w217:T11)  [unwired: 5 in, 1 out]
              n132 = local write "Additional floorspace\nfor second handler"(w226) -> ()
              n133 = call-poly <userlib>:"manageConfig.vi"("error in (no error)"=w207, "config ref"=w217) -> ()  [unwired: 9 in, 1 out]
            }
            frame #3 {
              w259 = "SCS.Notification.Enable text notification"  # key
              w265 = "SCS.Notification.Phone Number"  # key
              w266 = "SCS.Notification.Enable email notification"  # key
              w273 = "SCS.Notification.Email alert - Engineer"  # key
              # "Load data from the INI file for the Benefits tab"
              n134 = local read "Configuration file path and filename"() -> (w270:path)
              n135 = call-poly <userlib>:"manageConfig.vi"() -> ("error out"=w255:errorcluster, "config ref out"=w271:T11)  [unwired: 10 in]
              n136 = call-poly <userlib>:"manageConfig.vi"("error in (no error)"=w255, "access (0:read/write)"=enum16{"read/write", "read-only", "write-only"}."read-only", "config file path"=w270, "config ref"=w271) -> ("error out"=w254:errorcluster, "config ref out"=w274:T11)  [unwired: 5 in, 1 out]
              n137 = call-poly <userlib>:"manageConfig.vi"("error in"=w254, "property path"=w273, "config ref"=w274) -> ("error out"=w253:errorcluster, "value"=w268:string, "config ref out"=w264:T11)  [unwired: 5 in, 1 out]
              n138 = local write "Email alert - engineer"(w268) -> ()
              n139 = call-poly <userlib>:"manageConfig.vi"("error in"=w253, "property path"="SCS.Notification.Email alert CC", "config ref"=w264) -> ("error out"=w252:errorcluster, "value"=w267:string, "config ref out"=w263:T11)  [unwired: 5 in, 1 out]
              n140 = local write "Email alert - CC"(w267) -> ()
              n141 = call-poly <userlib>:"manageConfig.vi"("error in"=w252, "property path"=w266, "config ref"=w263) -> ("error out"=w251:errorcluster, "value"=w261:bool, "config ref out"=w258:T11)  [unwired: 5 in, 1 out]
              n142 = local write "Enable email notification"(w261) -> ()
              n143 = call-poly <userlib>:"manageConfig.vi"("error in"=w251, "property path"=w259, "config ref"=w258) -> ("error out"=w250:errorcluster, "value"=w256:bool, "config ref out"=w257:T11)  [unwired: 5 in, 1 out]
              n144 = local write "Enable text notification"(w256) -> ()
              n145 = call-poly <userlib>:"manageConfig.vi"("error in"=w250, "property path"=w265, "config ref"=w257) -> ("error out"=w249:errorcluster, "value"=w260:string, "config ref out"=w262:T11)  [unwired: 5 in, 1 out]
              n146 = local write "Phone number"(w260) -> ()
              n147 = call-poly <userlib>:"manageConfig.vi"("error in (no error)"=w249, "config ref"=w262) -> ()  [unwired: 9 in, 1 out]
            }
            frame #4 {
              # "This reads the GPIB addresses and related command from the INI file (.cfg)"
              n148 = local read "Configuration file path and filename"() -> (w301:path)
              n149 = call-poly <userlib>:"manageConfig.vi"() -> ("config ref out"=w302:T11)  [unwired: 10 in, 1 out]
              n150 = call-poly <userlib>:"manageConfig.vi"("access (0:read/write)"=enum16{"read/write", "read-only", "write-only"}."read-only", "config file path"=w301, "config ref"=w302) -> ("error out"=w304:errorcluster, "config ref out"=w306:T11)  [unwired: 6 in, 1 out]
              n151 = call-poly <userlib>:"manageConfig.vi"("error in"=w304, "property path"="SCS.GPIB.Tester Address" ("key"), "config ref"=w306) -> ("error out"=w291:errorcluster, "value"=w283:string, "config ref out"=w297:T11)  [unwired: 5 in, 1 out]
              n152 = local write "Tester address"(w283) -> ()
              n153 = call-poly <userlib>:"manageConfig.vi"("error in"=w291, "property path"="SCS.GPIB.H1 Address" ("key"), "config ref"=w297) -> ("error out"=w290:errorcluster, "value"=w282:string, "config ref out"=w296:T11)  [unwired: 5 in, 1 out]
              n154 = local write "H1 Address"(w282) -> ()
              n155 = call-poly <userlib>:"manageConfig.vi"("error in"=w290, "property path"="SCS.GPIB.H2 Address" ("key"), "config ref"=w296) -> ("error out"=w289:errorcluster, "value"=w281:string, "config ref out"=w295:T11)  [unwired: 5 in, 1 out]
              n156 = local write "H2 Address"(w281) -> ()
              n157 = call-poly <userlib>:"manageConfig.vi"("error in"=w289, "property path"="SCS.GPIB.SOT" ("key"), "config ref"=w295) -> ("error out"=w288:errorcluster, "config ref out"=w277:T11)  [unwired: 5 in, 2 out]
              n158 = call-poly <userlib>:"manageConfig.vi"("error in"=w288, "property path"="SCS.GPIB.Get Handler Velocity" ("key"), "config ref"=w277) -> ("error out"=w287:errorcluster, "value"=w280:string, "config ref out"=w276:T11)  [unwired: 5 in, 1 out]
              n159 = local write "Get Handler Velocity"(w280) -> ()
              n160 = call-poly <userlib>:"manageConfig.vi"("error in"=w287, "property path"="SCS.GPIB.Increase Handler Velocity" ("key"), "config ref"=w276) -> ("error out"=w286:errorcluster, "value"=w279:string, "config ref out"=w275:T11)  [unwired: 5 in, 1 out]
              n161 = local write "Increase Handler Velocity"(w279) -> ()
              n162 = call-poly <userlib>:"manageConfig.vi"("error in"=w286, "property path"="SCS.GPIB.Decrease Handler Velocity" ("key"), "config ref"=w275) -> ("error out"=w285:errorcluster, "value"=w278:string, "config ref out"=w284:T11)  [unwired: 5 in, 1 out]
              n163 = local write "Decrease Handler Velocity"(w278) -> ()
              n164 = call-poly <userlib>:"manageConfig.vi"("error in (no error)"=w285, "config ref"=w284) -> ()  [unwired: 9 in, 1 out]
            }
          }
        }
      }
    }
    frame #4 {
      # "This frame writes the headewr to the data log.\nIt includes setup and configuration information for the lot."
      n165 = local read "POWER"() -> (w307:bool)
      n166 = case shown="True" w307 {
        frame False {
        }
        frame True {
          w313 = "\r\n"
          n167 = local read "Lot number"() -> (w317:string)
          n168 = local read "Test cell ID"() -> (w315:string)
          n169 = local read "H1 online"() -> (w325:bool)
          n170 = local read "H2 online"() -> (w326:bool)
          n171 = local read "Data log path and filename"() -> (w308:path)
          n172 = local read "Operator name"() -> (w319:string)
          n173 = local read "H1 UPH warning limit hid"() -> (w321:dbl)
          n174 = local read "H2 UPH warning limit hid"() -> (w323:dbl)
          n175 = local read "H2  low yield warning"() -> (w322:dbl)
          n176 = local read "H1 low yield warning"() -> (w320:dbl)
          n177 = case shown="True" w325 {
            tunnel: ["H1 Off-Line" "H1 On-Line"] -> w327
            frame False {
            }
            frame True {
            }
          }
          n178 = case shown="True" w326 {
            tunnel: ["H2 Off-Line" "H2 On-Line"] -> w332
            frame False {
            }
            frame True {
            }
          }
          n179 = local write "Email alert - attachment (not editable)"(w308) -> ()
          n180 = Number To Decimal String(number=w320) -> (decimal integer string=w329:string)  [unwired: 1 in]
          n181 = Number To Decimal String(number=w321) -> (decimal integer string=w331:string)  [unwired: 1 in]
          n182 = Number To Decimal String(number=w322) -> (decimal integer string=w334:string)  [unwired: 1 in]
          n183 = Number To Decimal String(number=w323) -> (decimal integer string=w336:string)  [unwired: 1 in]
          n184 = Get Date/Time String() -> (date string=w310:string, time string=w312:string)  [unwired: 3 in]
          n185 = Concatenate Strings(w310, "   " ("string"), w312, w313, "Test Cell ID: ", w315, w313, "Lot Number: ", w317, w313, "Operator Name:  ", w319, w313, "System Started", w313, w327, w313, "H1 Low Yield Warning Limit: ", w329, w313, "H1 Low UPH Warning Limit: ", w331, w313, w332, w313, "H2 Low Yield Warning Limit: ", w334, w313, "H2 Low UPH Warning Limit: ", w336, w313, w313) -> (w337:string)
          n186 = call "SentinelDatalog.vi"("operation (0:open)"=T10."open or create", "String"=w337, "data log path"=w308) -> ()  [unwired: 8 in, 1 out]
        }
      }
    }
    frame #5 {
      # "This frame implements the main Sentinel Controller loop.\nAll loops within this frame execute as parallel processes."
      n187 = local read "POWER"() -> (w342:bool)
      n188 = case shown="True" w342 {
        frame False {
        }
        frame True {
          n189 = while {
            stop <- w357 stop-if-true
            w347 = 0
            w346 = 0.0
            w354 = 0
            w355 = 0.0
            # "Sentinel operating loop\n- tester loop\n- H1 loop\n- H2 loop\n- controls loop\n- alarm state machine loop\nExit with Power off"
            n190 = local read "POWER"() -> (w358:bool)
            n191 = Wait (ms)(milliseconds to wait=u32 100) -> ()  [unwired: 1 out]
            n192 = Not(x=w358) -> (.not. x?=w357:bool)
            n193 = while {
              i -> [w3125]
              stop <- w3141 stop-if-true
              n194 = local read "Run"() -> (w3117:bool)
              n195 = First Call?() -> (First Call?: T/F=w3118:bool)
              n196 = case shown="True" w3117 {
                frame False {
                  n197 = local write "Tester online"(FALSE ("Tester online")) -> ()
                  n198 = local write "H2 online"(FALSE ("H2 online")) -> ()
                  n199 = local write "H1 online"(FALSE ("H1 online")) -> ()
                }
                frame True {
                }
              }
              n200 = local read "Additional floorspace\nfor second handler"() -> (w3126:i32)
              n201 = Wait (ms)(milliseconds to wait=u32 50) -> ()  [unwired: 1 out]
              n202 = local read "Optimize handler speed"() -> (w3134:bool)
              n203 = local read "Std cell \nfloorspace area"() -> (w3139:i32)
              n204 = local read "Std cell \nfloorspace area"() -> (w3111:i32)
              n205 = local read "Celerint hardware cost ($/mo)"() -> (w3129:dbl)
              n206 = local read "Celerint licensing cost ($/mo)"() -> (w3128:dbl)
              n207 = local read "Second handler cost ($/mo)"() -> (w3127:dbl)
              n208 = case shown="True" w3118 {
                frame False {
                }
                frame True {
                  n209 = local read "H1 parallelism"() -> (w3174:u32)
                  n210 = local read "H2 parallelism"() -> (w3173:u32)
                  n211 = local read "H1 index time expected hid"() -> (w3172:dbl)
                  n212 = local read "H1 index time expected hid"() -> (w3182:dbl)
                  n213 = local read "H2 index time expected hid"() -> (w3171:dbl)
                  n214 = local read "H2 index time expected hid"() -> (w3183:dbl)
                  n215 = local read "Test time expected hid"() -> (w3180:dbl)
                  n216 = local write "H2 units/cycle"(w3173) -> ()
                  n217 = local write "H1 units/cycle"(w3174) -> ()
                  n218 = formula code="H1UPHorig=P1*3600/(T+H1ITorig);\nH2UPHorig=P2*3600/(T+H2ITorig);\nSYSH1WT=T-H1I;\nSYSH2WT=T-H2I;"("T"=w3180, "H1I"=w3172, "H2I"=w3171, "P1"=w3174, "H1ITorig"=w3182, "H2ITorig"=w3183, "P2"=w3173) -> ("H1UPHorig"=w3170:dbl, "H2UPHorig"=w3169:dbl, "SYSH1WT"=w3189:dbl, "SYSH2WT"=w3188:dbl)
                  n219 = local write "H1 Index Time 2"(w3172) -> ()
                  n220 = local write "H1 Test Time 2"(w3171) -> ()
                  n221 = local write "H1 P in formula"(w3174) -> ()
                  n222 = local write "H2 calc UPH"(w3169) -> ()
                  n223 = local read "H1 index time expected hid"() -> (w3176:dbl)
                  n224 = local read "H2 index time expected hid"() -> (w3175:dbl)
                  n225 = local read "Test time expected hid"() -> (w3177:dbl)
                  n226 = local write "H1 calc UPH"(w3170) -> ()
                  n227 = local write "UPH"(w3170) -> ()
                  n228 = local read "H2 parallelism"() -> (w3179:u32)
                  n229 = local read "H1 parallelism"() -> (w3178:u32)
                  n230 = Less Than 0?(x=w3189) -> (x < 0?=w3190:bool)
                  n231 = Less Than 0?(x=w3188) -> (x < 0?=w3191:bool)
                  n232 = Select(t=0.0, s=w3190, f=w3189) -> (s? t:f=w3185:dbl)
                  n233 = Select(t=0.0, s=w3191, f=w3188) -> (s? t:f=w3184:dbl)
                  n234 = local read "H1 index time expected hid"() -> (w3168:dbl)
                  n235 = local read "H2 index time expected hid"() -> (w3167:dbl)
                  n236 = local read "Test time expected hid"() -> (w3163:dbl)
                  n237 = formula code="ExpH1UPH=P1*3600/(T+SYSH1I+SYSH1WT);\nExpH2UPH=P2*3600/(T+SYSH2I+SYSH2WT);\nMaxUPH=Margin*(ExpH1UPH+ExpH2UPH);"("P1"=w3179, "T"=w3177, "SYSH1I"=w3176, "SYSH2I"=w3175, "Margin"=1.05 ("input variable"), "SYSH1WT"=w3185, "SYSH2WT"=w3184, "P2"=w3178) -> ("MaxUPH"=w3181:dbl, "ExpH1UPH"=w3187:dbl, "ExpH2UPH"=w3186:dbl)
                  n238 = Add(x=w3168, y=w3167) -> (x+y=w3166:dbl)
                  n239 = Divide(x=w3166, y=2.0) -> (x/y=w3164:dbl)
                  n240 = Add(x=w3163, y=w3164) -> (x+y=w3162:dbl)
                  n241 = Multiply(x=4000.0, y=w3162) -> (x*y=w3160:dbl)
                  n242 = To Unsigned Long Integer(number=w3160) -> (unsigned 32bit integer=w3159:u32)
                  n243 = local write "GPIB wait timeout hid"(w3159) -> ()
                  n244 = property on="System UPH" class="Knob (strict)"("Scale.Maximum"=w3181) -> ()  [unwired: 2 in, 2 out]
                  n245 = property on="H1 UPH" class="Knob (strict)"("Scale.Maximum"=w3187) -> ()  [unwired: 2 in, 2 out]
                  n246 = property on="H2 UPH" class="Knob (strict)"("Scale.Maximum"=w3186) -> ()  [unwired: 2 in, 2 out]
                }
              }
              n247 = local read "Handler cost ($/mo)"() -> (w3131:dbl)
              n248 = local read "Tester cost ($/mo)"() -> (w3132:dbl)
              n249 = local read "H1 online"() -> (w3121:bool)
              n250 = local read "H2 online"() -> (w3120:bool)
              n251 = local read "Overhead ($/mo)"() -> (w3130:dbl)
              n252 = local read "POWER"() -> (w3143:bool)
              n253 = Not(x=w3143) -> (.not. x?=w3142:bool)
              n254 = Not(x=w3121) -> (.not. x?=w3109:bool)
              n255 = Not(x=w3120) -> (.not. x?=w3108:bool)
              n256 = local read "Hours per month"() -> (w3113:i32)
              n257 = case shown="True" w3134 {
                frame False {
                }
                frame True {
                  # "place code here to optimize handler index times"
                }
              }
              n258 = local write "Std cell floorspace area"(w3111) -> ()
              n259 = Compound Arithmetic op=OR(w3142) -> (w3141:bool)
              n260 = And(x=w3109, y=w3108) -> (x .and. y?=w3119:bool)
              n261 = case shown="True" w3109 {
                frame False {
                }
                frame True {
                  n262 = local write "H1 nominal 2"(TRUE) -> ()
                  n263 = local write "H1 nominal"(TRUE) -> ()
                  n264 = local write "H1 warning 2"(TRUE) -> ()
                  n265 = local write "H1 warning"(TRUE) -> ()
                  n266 = local write "H1 alarm 2"(TRUE) -> ()
                  n267 = local write "H1 alarm"(TRUE) -> ()
                }
              }
              n268 = local write "H1 On/Off-line"(w3109) -> ()
              n269 = case shown="True" w3108 {
                frame False {
                }
                frame True {
                  n270 = local write "H2 nominal"(TRUE) -> ()
                  n271 = local write "H2 nominal 2"(TRUE) -> ()
                  n272 = local write "H2 warning"(TRUE) -> ()
                  n273 = local write "H2 warning 2"(TRUE) -> ()
                  n274 = local write "H2 alarm"(TRUE) -> ()
                  n275 = local write "H2 alarm 2"(TRUE) -> ()
                }
              }
              n276 = local write "H2 On/Off-line"(w3108) -> ()
              n277 = Add(x=w3126, y=w3139) -> (x+y=w3110:i32)
              n278 = Compound Arithmetic op=ADD(w3132, w3131, w3130) -> (w3136:dbl)
              n279 = Compound Arithmetic op=ADD(w3129, w3128, w3127) -> (w3137:dbl)
              n280 = Compound Arithmetic op=ADD(w3132, w3130) -> (w3114:dbl)
              n281 = case shown="False" w3119 {
                frame False {
                }
                frame True {
                  n282 = local write "System UPH"(u32 0 ("System UPH")) -> ()
                  n283 = local write "Sys utilization"(0.0 ("Sys utilization")) -> ()
                }
              }
              n284 = local write "Tandem\nfloorspace area"(w3110) -> ()
              n285 = Divide(x=w3137, y=w3113) -> (x/y=w3140:dbl)
              n286 = Add(x=w3137, y=w3136) -> (x+y=w3116:dbl)
              n287 = Divide(x=w3136, y=w3113) -> (x/y=w3112:dbl)
              n288 = local write "Hours per month 2"(w3113) -> ()
              n289 = local write "Total Mo Costs ($/mo) 2"(w3114) -> ()
              n290 = local write "Total Mo Costs ($/mo) 3"(w3116) -> ()
              n291 = local write "Std mo cost ($/mo)"(w3114) -> ()
              n292 = Add(x=w3112, y=w3140) -> (x+y=w3115:dbl)
              n293 = local write "Std hourly\ncost ($/hr)"(w3112) -> ()
              n294 = local read "Push to reset charts"() -> (w3123:bool)
              n295 = local write "Tandem hourly\ncost ($/hr)"(w3115) -> ()
              n296 = local read "Optimize handler speed"() -> (w3122:bool)
              n297 = case shown="True" w3123 {
                frame False {
                }
                frame True {
                  n298 = property on="YieldMon" class="WFChart (strict)"("History Data"=cluster{dbl, dbl, dbl, dbl}[] [{100.0, 100.0, 0.0, 0.0}]) -> ()  [unwired: 2 in, 2 out]
                  n299 = property on="SysUtilMon" class="WFChart (strict)"("History Data"=cluster{dbl, dbl}[] []) -> ()  [unwired: 2 in, 2 out]
                }
              }
              n300 = Equal To 0?(x=w3125) -> (x = 0?=w3124:bool)
              n301 = case shown="True" w3124 {
                frame False {
                }
                frame True {
                  w3218 = "" ("Message from tester")
                  w3221 = 0
                  w3224 = 0
                  w3237 = 100
                  w3238 = 0
                  w3239 = FALSE ("H1 alarm")
                  # "graphs and charts - declared here, displayed elsewhere"
                  n302 = Bundle(w3237, w3237, w3237, w3237) -> (w3216:cluster{i32, i32, i32, i32})  [unwired: 1 in]
                  n303 = Bundle(w3238, w3238) -> (w3215:cluster{i32, i32})  [unwired: 1 in]
                  n304 = local write "H2 Lock"(FALSE ("H2 Lock")) -> ()
                  n305 = local write "H1 alarm"(FALSE ("H1 warning")) -> ()
